vi "公式节点.vi"() -> ()   [LabVIEW 2017]
panel:
  out "波形图":dbl[][](graph)
  out "y2":dbl
  out "y1":dbl
  in  "b":dbl
  in  "a":dbl
  in  "x":dbl
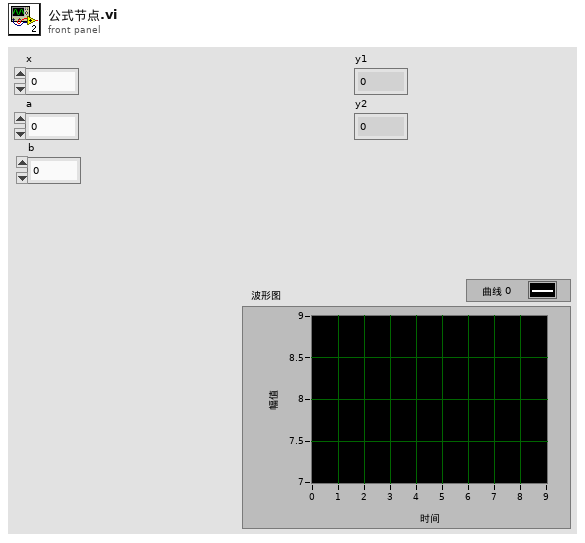
[diagram p1: front panel]
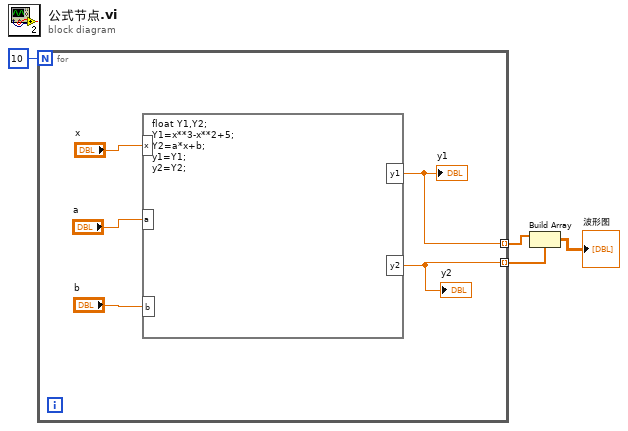
[diagram p0: block diagram]
diagram:
  n1 = for {
    N: 10 -> [_]
    tunnel: [w6] -> w4 mode=indexing
    tunnel: [w5] -> w3 mode=indexing
    n2 = formula code="float Y1,Y2;\nY1=x**3-x**2+5;\nY2=a*x+b;\ny1=Y1;\ny2=Y2;"("x"="x", "a"="a", "b"="b") -> ("y1"=w6:dbl, "y2"=w5:dbl)
    "y1" <- w6
    "y2" <- w5
  }
  n3 = Build Array(w4, w3) -> (→"波形图":dbl[][])
